vi "Teleop.vi"(10 "Match Info":T1={"Autonomous Elapsed Seconds"=0.0, "TeleOp Elapsed Seconds"=0.0, "Disabled Elapsed Seconds"=0.0, "Visited Autonomous"=FALSE, "Visited TeleOp"=FALSE, "Visited Disabled"=FALSE, "Autonomous Settings"={"Autonomous Style"=enum."Independent", "VI Refnum"=refnum}}, 11 "Call Context":T2) -> ()   [LabVIEW 2017]
doc: "This VI is called for each TeleOp packet received from the DS where the robot is not disabled. It is often used to read from the joysticks and update I/O or to update setpoints for timed control loops. It should complete and return within 20 milliseconds or it may miss DS packets."
uses:
  <vilib>/Rock Robotics/WPI/DriverStation/WPI_DriverStationDerivedRobotMode.ctl
  <vilib>/Rock Robotics/WPI/DriverStation/WPI_DriverStationMatch Info.ctl
  CommandTypes/LiftCommands.ctl
  CommandTypes/IntakeCommands.ctl
  CommandTypes/DriveCommands.ctl
  <vilib>/Rock Robotics/WPI/Utilities/WPI_GetSetVariantRefNum.vi
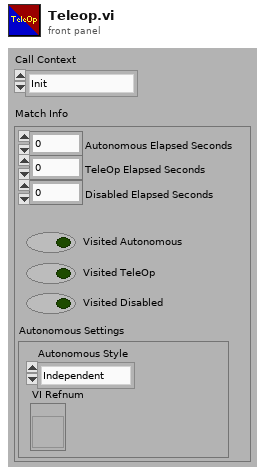
[diagram p1: front panel]
types:
  T1 = typedef "WPI_DriverStationMatch Info.ctl" = cluster{"Autonomous Elapsed Seconds":dbl, "TeleOp Elapsed Seconds":dbl, "Disabled Elapsed Seconds":dbl, "Visited Autonomous":bool, "Visited TeleOp":bool, "Visited Disabled":bool, "Autonomous Settings":cluster{"Autonomous Style":enum16{"Iterative", "Independent"}, "VI Refnum":refnum<vi>}}
  T2 = typedef "WPI_DriverStationDerivedRobotMode.ctl" = enum16{"Init", "Execute", "Stop"}
  T3 = typedef "WPI_JoystickDevRef.ctl" = cluster{"Device":T4}
  T4 = typedef "WPI_JoystickDeviceEnum.ctl" = enum16{"USB 0", "USB 1", "USB 2", "USB 3", "USB 4", "USB 5"}
  T5 = typedef "IntakeCommands.ctl" = enum16{"Do Nothing", "Manuel", "Score", "Acquire"}
  T6 = typedef "LiftCommands.ctl" = enum16{"Do  Nothing", "Manuel", "Home", "Ground", "To Switch", "To Scale Low", "To Scale Medium", "To Scale High"}
  T7 = typedef "DriveCommands.ctl" = enum16{"Center on Cube", "Manual", "Acquire Cube", "Drive Path"}
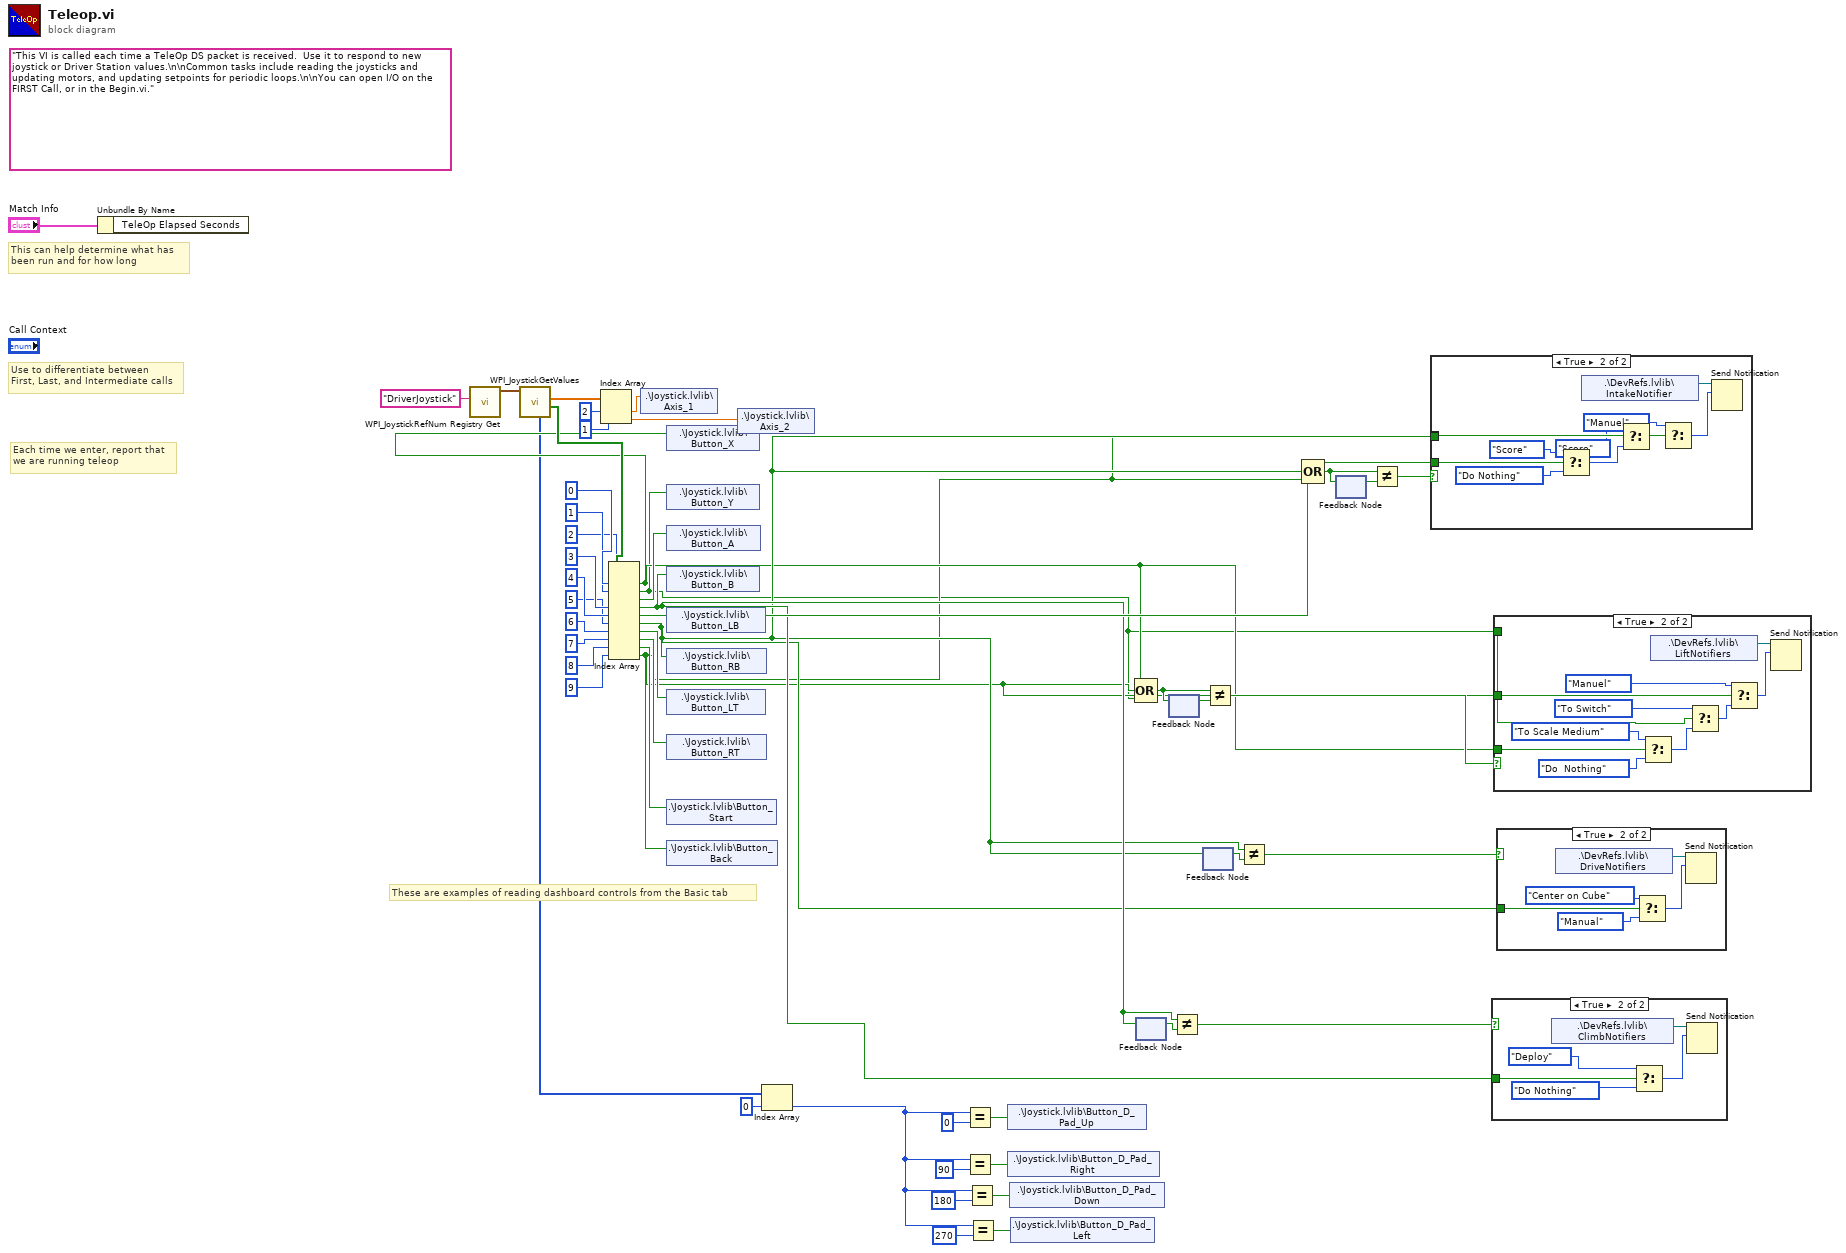
[diagram p0: block diagram]
diagram:
  (unwired) "This VI is called each time a TeleOp DS packet is received.  Use it to respond to new joystick or Driver Station values.\n\nCommon tasks include reading the joysticks and updating motors, and updating setpoints for periodic loops.\n\nYou can open I/O on the FIRST Call, or in the Begin.vi."
  # "These are examples of reading dashboard controls from the Basic tab"
  # "Each time we enter, report that\nwe are running teleop"
  # "Use to differentiate between\nFirst, Last, and Intermediate calls"
  # "This can help determine what has\nbeen run and for how long"
  n1 = Unbundle By Name("Match Info") -> ()  [unwired: 1 out]
  n2 = call <vilib>:"WPI_JoystickRefNum Registry Get.vi"("refnum name"="DriverJoystick") -> ("JoystickDevRef"=w49:T3)  [unwired: 1 in, 9 out]
  n3 = call <vilib>:"WPI_JoystickGetValues.vi"("JoystickDevRef"=w49) -> ("Buttons"=w46:bool[], "Axes"=w48:dbl[], "POVs"=w11:i16[])  [unwired: 6 in, 2 out]
  n4 = Index Array(array=w48, index #1=2 ("index"), index #2=1 ("index")) -> (element #1=w45:dbl, element #2=w44:dbl)
  n5 = Index Array(array=w46, index #1=0 ("index"), index #2=1 ("index"), index #3=2 ("index"), index #4=3 ("index"), index #5=4 ("index"), index #6=5 ("index"), index #7=6 ("index"), index #8=7 ("index"), index #9=8 ("index"), index #10=9 ("index")) -> (element #1=w14:bool, element #2=w12:bool, element #3=w28:bool, element #4=w21:bool, element #5=w27:bool, element #6=w18:bool, element #7=w30:bool, element #8=w31:bool, element #9=w29:bool, element #10=w13:bool)
  n6 = shared-variable ".\\Joystick.lvlib\\Axis_1"(w45) -> ()  [unwired: 1 in, 1 out]
  n7 = shared-variable ".\\Joystick.lvlib\\Button_X"(w14) -> ()  [unwired: 1 in, 1 out]
  n8 = shared-variable ".\\Joystick.lvlib\\Button_Y"(w12) -> ()  [unwired: 1 in, 1 out]
  n9 = shared-variable ".\\Joystick.lvlib\\Button_A"(w28) -> ()  [unwired: 1 in, 1 out]
  n10 = shared-variable ".\\Joystick.lvlib\\Button_B"(w21) -> ()  [unwired: 1 in, 1 out]
  n11 = shared-variable ".\\Joystick.lvlib\\Button_LB"(w27) -> ()  [unwired: 1 in, 1 out]
  n12 = shared-variable ".\\Joystick.lvlib\\Button_RB"(w18) -> ()  [unwired: 1 in, 1 out]
  n13 = shared-variable ".\\Joystick.lvlib\\Button_LT"(w30) -> ()  [unwired: 1 in, 1 out]
  n14 = shared-variable ".\\Joystick.lvlib\\Button_RT"(w31) -> ()  [unwired: 1 in, 1 out]
  n15 = shared-variable ".\\Joystick.lvlib\\Button_Start"(w29) -> ()  [unwired: 1 in, 1 out]
  n16 = shared-variable ".\\Joystick.lvlib\\Button_Back"(w13) -> ()  [unwired: 1 in, 1 out]
  n17 = shared-variable ".\\Joystick.lvlib\\Axis_2"(w44) -> ()  [unwired: 1 in, 1 out]
  n18 = Index Array(array=w11, index=0) -> (element=w5:i16)
  n19 = Equal?(x=w5, y=i16 0) -> (x = y?=w9:bool)
  n20 = Equal?(x=w5, y=i16 90) -> (x = y?=w8:bool)
  n21 = Equal?(x=w5, y=i16 180) -> (x = y?=w7:bool)
  n22 = Equal?(x=w5, y=i16 270) -> (x = y?=w6:bool)
  n23 = shared-variable ".\\Joystick.lvlib\\Button_D_Pad_Up"(w9) -> ()  [unwired: 1 in, 1 out]
  n24 = shared-variable ".\\Joystick.lvlib\\Button_D_Pad_Right"(w8) -> ()  [unwired: 1 in, 1 out]
  n25 = shared-variable ".\\Joystick.lvlib\\Button_D_Pad_Down"(w7) -> ()  [unwired: 1 in, 1 out]
  n26 = shared-variable ".\\Joystick.lvlib\\Button_D_Pad_Left"(w6) -> ()  [unwired: 1 in, 1 out]
  n27 = Compound Arithmetic op=OR(w14, w13, w12) -> (w15:bool)
  n28 = feedback #1() -> (w23:bool)  [unwired: 1 in]
  n29 = feedback-in #1(w21) -> ()
  n30 = feedback #2() -> (w17:bool)  [unwired: 1 in]
  n31 = feedback-in #2(w15) -> ()
  n32 = Not Equal?(x=w21, y=w23) -> (x != y?=w22:bool)
  n33 = feedback #3() -> (w20:bool)  [unwired: 1 in]
  n34 = feedback-in #3(w18) -> ()
  n35 = Not Equal?(x=w15, y=w17) -> (x != y?=w16:bool)
  n36 = Not Equal?(x=w18, y=w20) -> (x != y?=w19:bool)
  n37 = Compound Arithmetic op=OR(w27, w18, w13) -> (w24:bool)
  n38 = feedback-in #4(w24) -> ()
  n39 = feedback #4() -> (w25:bool)  [unwired: 1 in]
  n40 = Not Equal?(x=w24, y=w25) -> (x != y?=w26:bool)
  n41 = case shown="True" w26 {
    tunnel: w13 -> [_ w61]
    tunnel: w18 -> [_ w60]
    tunnel: w27 -> [_ w59]
    frame False {
    }
    frame True {
      n42 = Select(t=IntakeCommands."Score", s=w59, f=IntakeCommands."Do Nothing") -> (s? t:f=w54:T5)
      n43 = shared-variable ".\\DevRefs.lvlib\\IntakeNotifier"() -> (w58:refnum<notifier>)  [unwired: 1 in, 1 out]
      n44 = Select(t=IntakeCommands."Score", s=w60, f=w54) -> (s? t:f=w55:T5)
      n45 = Select(t=IntakeCommands."Manuel", s=w61, f=w55) -> (s? t:f=w57:T5)
      n46 = Send Notification(notification=w57, notifier=w58) -> ()  [unwired: 1 in, 2 out]
    }
  }
  n47 = case shown="True" w22 {
    tunnel: w21 -> [_ w66]
    frame False {
    }
    frame True {
      n48 = shared-variable ".\\DevRefs.lvlib\\ClimbNotifiers"() -> (w65:refnum<notifier>)  [unwired: 1 in, 1 out]
      n49 = Select(t=enum16{"Do Nothing", "Deploy"}."Deploy" ("Enum"), s=w66, f=enum16{"Do Nothing", "Deploy"}."Do Nothing" ("Enum")) -> (s? t:f=w64:enum16{"Do Nothing", "Deploy"})
      n50 = Send Notification(notification=w64, notifier=w65) -> ()  [unwired: 1 in, 2 out]
    }
  }
  n51 = case shown="True" w16 {
    tunnel: w13 -> [_ w77]
    tunnel: w14 -> [_ w73]
    tunnel: w12 -> [_ w72]
    frame False {
    }
    frame True {
      n52 = Select(t=LiftCommands."To Scale Medium" ("notification"), s=w73, f=LiftCommands."Do  Nothing" ("notification")) -> (s? t:f=w74:T6)
      n53 = shared-variable ".\\DevRefs.lvlib\\LiftNotifiers"() -> (w76:refnum<notifier>)  [unwired: 1 in, 1 out]
      n54 = Select(t=LiftCommands."To Switch" ("notification"), s=w72, f=w74) -> (s? t:f=w75:T6)
      n55 = Select(t=LiftCommands."Manuel" ("notification"), s=w77, f=w75) -> (s? t:f=w71:T6)
      n56 = Send Notification(notification=w71, notifier=w76) -> ()  [unwired: 1 in, 2 out]
    }
  }
  n57 = case shown="True" w19 {
    tunnel: w18 -> [_ w82]
    frame False {
    }
    frame True {
      n58 = shared-variable ".\\DevRefs.lvlib\\DriveNotifiers"() -> (w81:refnum<notifier>)  [unwired: 1 in, 1 out]
      n59 = Select(t=DriveCommands."Center on Cube", s=w82, f=DriveCommands."Manual") -> (s? t:f=w78:T7)
      n60 = Send Notification(notification=w78, notifier=w81) -> ()  [unwired: 1 in, 2 out]
    }
  }
